vi "finalX.vi"(10 "Momentum [MeV/C](pixel)":dbl[](array[numeric]), 11 "intraY":dbl) -> (2 "finalX":dbl[][](array[numeric]))   [LabVIEW 2013]
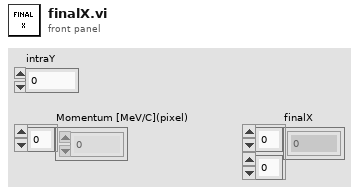
[diagram p1: front panel]
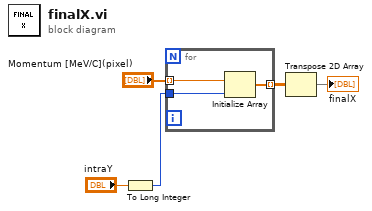
[diagram p0: block diagram]
diagram:
  n1 = To Long Integer(number="intraY") -> (32bit integer=w1:i32)
  n2 = for {
    tunnel: "Momentum [MeV/C](pixel)" -> [w8] mode=indexing
    tunnel: w1 -> [w7]
    tunnel: [w6] -> w2 mode=indexing
    n3 = Initialize Array(w8, w7) -> (w6:dbl[])
  }
  n4 = Transpose 2D Array(2D array=w2) -> (transposed array=→"finalX":dbl[][])
